vi "NoParent_ReturnsEmptyTag.vi"() -> (0 "error out":errorcluster)   [LabVIEW 2017, in "ResultTree.Tests.lvlib" / "GetParent.lvlib"]
uses:
  GetParent.lvlib
  2a6c7ef5-d8ea-4de4-ba7d-c6663dbf2225.vi
  Constraint/IsEqual/Create.vi
  Constraint/IsEqual/IsEqual.lvclass
  ResultTree/ResultTree.lvclass
panel:
  in  "Tree":string(tree)
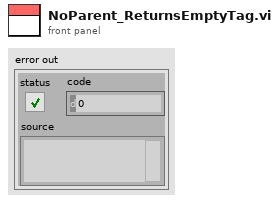
[diagram p1: front panel]
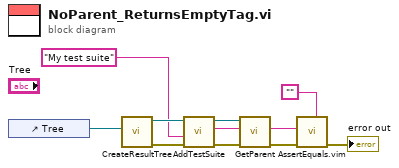
[diagram p0: block diagram]
diagram:
  n1 = control-ref of="Tree"() -> (w10:refnum<vi>)
  n2 = call "CreateResultTree.vi"("Tree Refnum"=w10) -> ("error out"=w9:errorcluster, "ResultTree out"=w8:refnum<class "ResultTree.lvclass">)  [unwired: 9 in]
  n3 = call "AddTestSuite.vi"("error in (no error)"=w9, "Name"="My test suite", "ResultTree in"=w8) -> ("error out"=w6:errorcluster, "Tag Name"=w3:string, "ResultTree out"=w2:refnum<class "ResultTree.lvclass">)  [unwired: 6 in]
  n4 = call "GetParent.vi"("error in (no error)"=w6, "Tag"=w3, "ResultTree in"=w2) -> ("error out"=w4:errorcluster, "Parent Tag"=w1:string)  [unwired: 6 in, 1 out]
  n5 = call "AssertEquals.vim"("Expected"="", "error in (no error)"=w4, "Actual"=w1) -> ("error out"=→"error out":errorcluster)  [unwired: 8 in]
